vi "PTScanner.check edit object.vi"(0 "Object cmds":T1[](array[typedef]), 2 "index":i32, 4 "new obj command":T1, 5 "error in (no error)":errorcluster) -> (14 "Object cmds out":T1[](array[typedef]), 19 "error out":errorcluster)   [LabVIEW 2014, in "PTScanner.lvlib"]
uses:
  PTScanner.lvlib
  PTScanner.obj parameters.ctl
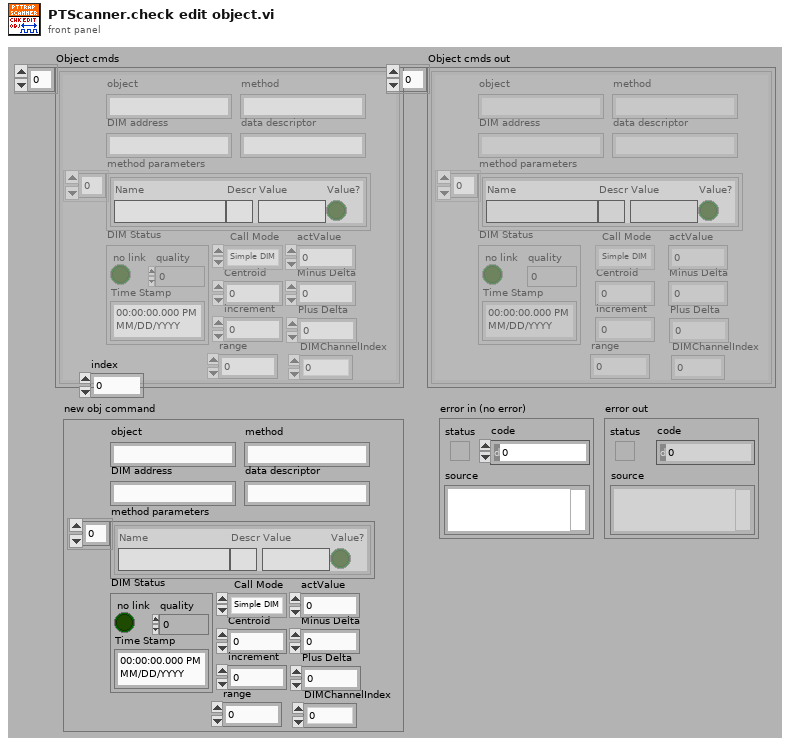
[diagram p1: front panel]
types:
  T1 = typedef "PTScanner.lvlib/PTScanner.obj parameters.ctl" = cluster{"object":string, "DIM address":string, "method":string, "data descriptor":string, "method parameters":cluster{"Name":string, "Descr":string, "Value":string, "Value?":bool}[], "Call Mode":enum16{"Simple DIM", "Synchronous"}, "actValue":dbl, "Centroid":dbl, "Minus Delta":dbl, "Plus Delta":dbl, "increment":dbl, "DIM Status":cluster{"no link":bool, "quality":i32, "Time Stamp":timestamp}, "range":dbl, "DIMChannelIndex":i32}
  T2 = cluster{"Name":string, "Descr":string, "Value":string, "Value?":bool}[]
  T3 = cluster{"object":string, "method":string, bool[]}
  T4 = cluster{"object":string, "method":string, bool[]}[]
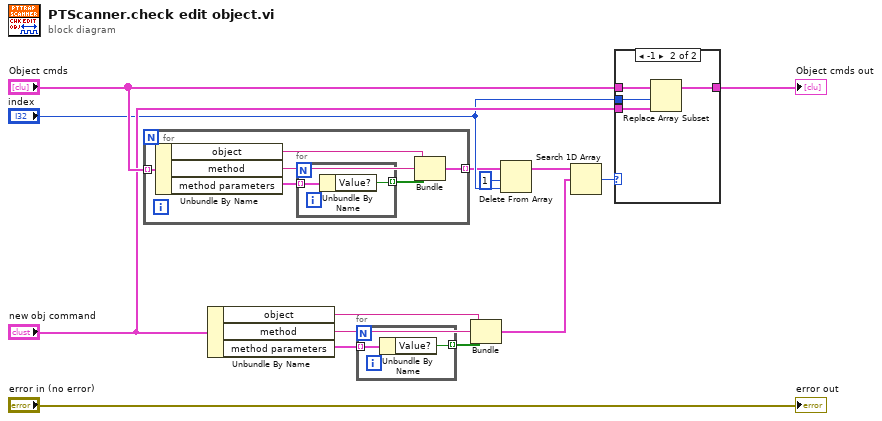
[diagram p0: block diagram]
diagram:
  n1 = for {
    tunnel: "Object cmds" -> [w20] mode=indexing
    tunnel: [w15] -> w3 mode=indexing
    n2 = Unbundle By Name(w20) -> ("object"=w18:string, "method"=w17:string, "method parameters"=w19:T2)
    n3 = for {
      tunnel: w19 -> [w21] mode=indexing
      tunnel: [w22] -> w16 mode=indexing
      n4 = Unbundle By Name(w21) -> ("Value?"=w22:bool)
    }
    n5 = Bundle("object"=w18, "method"=w17, w16) -> (w15:T3)  [unwired: 1 in]
  }
  n6 = Unbundle By Name("new obj command") -> ("object"=w8:string, "method"=w7:string, "method parameters"=w9:T2)
  n7 = for {
    tunnel: w9 -> [w24] mode=indexing
    tunnel: [w23] -> w6 mode=indexing
    n8 = Unbundle By Name(w24) -> ("Value?"=w23:bool)
  }
  n9 = Bundle("object"=w8, "method"=w7, w6) -> (w5:T3)  [unwired: 1 in]
  n10 = Delete From Array(array=w3, length=1, index="index") -> (array with subset deleted=w1:T4)  [unwired: 1 out]
  n11 = Search 1D Array(1D array=w1, element=w5) -> (index of element=w4:i32)  [unwired: 1 in]
  n12 = case shown="-1" w4 {
    tunnel: "Object cmds" -> [w25 w29]
    tunnel: [w25 w28] -> w12
    tunnel: "new obj command" -> [_ w27]
    tunnel: "index" -> [_ w26]
    frame 0, Default {
    }
    frame -1 {
      n13 = Replace Array Subset(array=w29, new element=w27, index=w26) -> (w28:T1[])
    }
  }
  "Object cmds out" <- w12
  "error out" <- "error in (no error)"
